vi "DAC Configure.vi"(8 "error in":errorcluster, 11 "DAC RTD Temp in":refnum<class "DAC RTD Temp.lvclass">) -> (0 "error out":errorcluster, 3 "DAC RTD Temp out":refnum<class "DAC RTD Temp.lvclass">)   [LabVIEW 2019, in "DAC.lvlib" / "DAC RTD Temp.lvclass"]
uses:
  DAC RTD Temp.lvclass
  DAC.lvclass
  C:/Users/wg/Documents/LV_Projects/test-stand/App/DAC/DAC.lvclass
  <vilib>/DAQmx/create/channels.llb/DAQmx Create Channel (AI-Temperature-RTD).vi
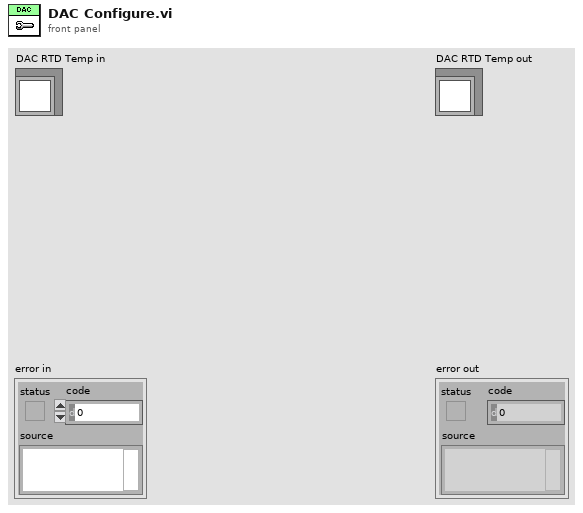
[diagram p1: front panel]
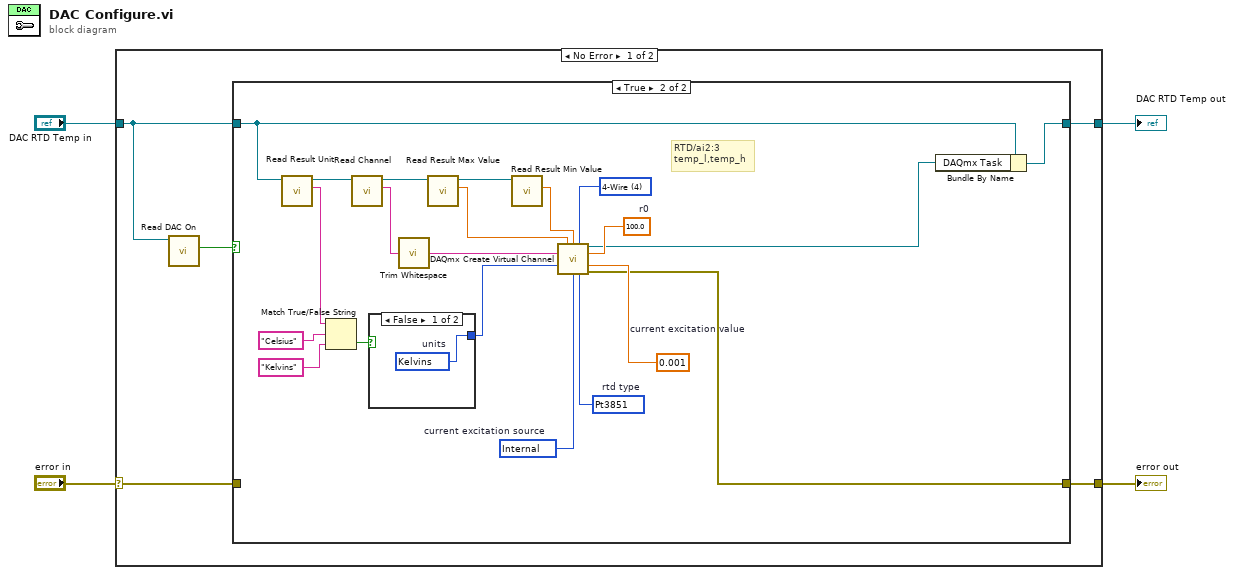
[diagram p0: block diagram]
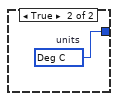
[diagram p3: hidden frame]
diagram:
  n1 = case shown="No Error" "error in" {
    selector: "error in" -> [w6 w36]
    tunnel: [w5 w36] -> w4
    tunnel: [w7 w35] -> w3
    tunnel: "DAC RTD Temp in" -> [w9 w35]
    frame No Error {
      n2 = call "Read DAC On.vi"("DAC in"=w9) -> ("DAC On"=w8:bool)  [unwired: 8 in, 2 out]
      n3 = case shown="True" w8 {
        tunnel: w9 -> [w11 w20]
        tunnel: [w11 w32] -> w7
        tunnel: w6 -> [w10 _]
        tunnel: [w10 w12] -> w5
        frame False {
        }
        frame True {
          w26 = 0.001  # current excitation value
          w27 = 10071 items=["Pt3750"=12481, "Pt3851"=10071, "Pt3911"=12482, "Pt3916"=10069, "Pt3920"=10053, "Pt3928"=12483, "Custom"=10137]  # rtd type
          w28 = 10200 items=["Internal"=10200, "External"=10167, "None"=10230]  # current excitation source
          w29 = 100.0  # r0
          w30 = 4 items=["2-Wire"=2, "3-Wire"=3, "4-Wire"=4] ("resistance configuration")
          # "RTD/ai2:3\ntemp_l,temp_h"
          n4 = call "Read Result Unit.vi"("DAC in"=w20) -> ("Unit"=w21:string, "DAC out"=w16:refnum<class "DAC RTD Temp.lvclass">)  [unwired: 8 in, 1 out]
          n5 = Match True/False String(2:"Kelvins" ("false string"), 3:"Celsius" ("true string"), 4:w21) -> (0:w22:bool)  [unwired: 1 out]
          n6 = call "Read Channel.vi"("DAC in"=w16) -> ("Channel"=w31:string, "DAC out"=w17:refnum<class "DAC RTD Temp.lvclass">)  [unwired: 8 in, 1 out]
          n7 = case shown="False" w22 {
            tunnel: [w33 w34] -> w19
            frame False {
              w33 = 10325 items=["Deg C"=10143, "Deg F"=10144, "Kelvins"=10325, "Deg R"=10145, "From Custom Scale"=10065]  # units
            }
            frame True {
              w34 = 10143 items=["Deg C"=10143, "Deg F"=10144, "Kelvins"=10325, "Deg R"=10145, "From Custom Scale"=10065]  # units
            }
          }
          n8 = call <vilib>:"Trim Whitespace.vi"("string"=w31) -> ("trimmed string"=w25:string)  [unwired: 1 in]
          n9 = call "Read Result Max Value.vi"("DAC in"=w17) -> ("Max Value"=w15:dbl, "DAC out"=w18:refnum<class "DAC RTD Temp.lvclass">)  [unwired: 8 in, 1 out]
          n10 = call "Read Result Min Value.vi"("DAC in"=w18) -> ("Min Value"=w14:dbl)  [unwired: 8 in, 2 out]
          n11 = call-poly <vilib>:"DAQmx Create Virtual Channel.vi"("maximum value"=w15, "minimum value"=w14, "resistance configuration"=w30, "physical channels"=w25, "r0"=w29, "units"=w19, "current excitation value"=w26, "current excitation source"=w28, "rtd type"=w27) -> ("task out"=w13:refnum<k21>, "error out"=w12:errorcluster)  [unwired: 5 in]
          n12 = Bundle By Name(cluster=w20, "DAQmx Task"=w13) -> (w32:refnum<class "DAC RTD Temp.lvclass">)
        }
      }
    }
    frame Error {
    }
  }
  "error out" <- w4
  "DAC RTD Temp out" <- w3
